vi "start_sweep.vi"(8 "error in (no error)":errorcluster, 11 "DL090430TriggeredExperimentController in":refnum<class "ExperimentControllerDL090803Triggered.lvclass">) -> (0 "error out":errorcluster, 3 "DL090430TriggeredExperimentController out":refnum<class "ExperimentControllerDL090803Triggered.lvclass">)   [LabVIEW 2010, in "ExperimentControllerDL090803Triggered.lvclass"]
uses:
  ExperimentControllerDL090803Triggered.lvclass
  ExperimentControllerDL090803Triggered.lvclass/ExperimentControllerDL090803Triggered.ctl
  DAQ/GenericDAQ/GenericDAQ/GenericDAQ.lvclass
  ScanHead/GenericScanHead/GenericScanHead/GenericScanHead.lvclass
  ImagingMode/GenericImagingMode/GenericImagingMode/GenericImagingMode.lvclass
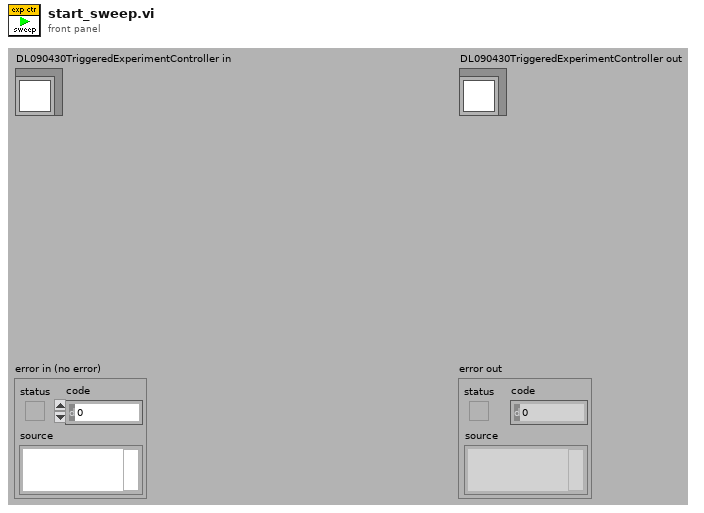
[diagram p1: front panel]
types:
  T1 = typedef "GenericToplevelComponent.lvclass/common_trigger_enum.ctl" = enum16{"NULL", "initialise", "terminate", "fetch command", "fetch data", "attach observer", "register as observer", "detach observer", "acknowledge", "start", "stop", "sweep started", "sweep finished", "experiment started", "experiment stopped"}
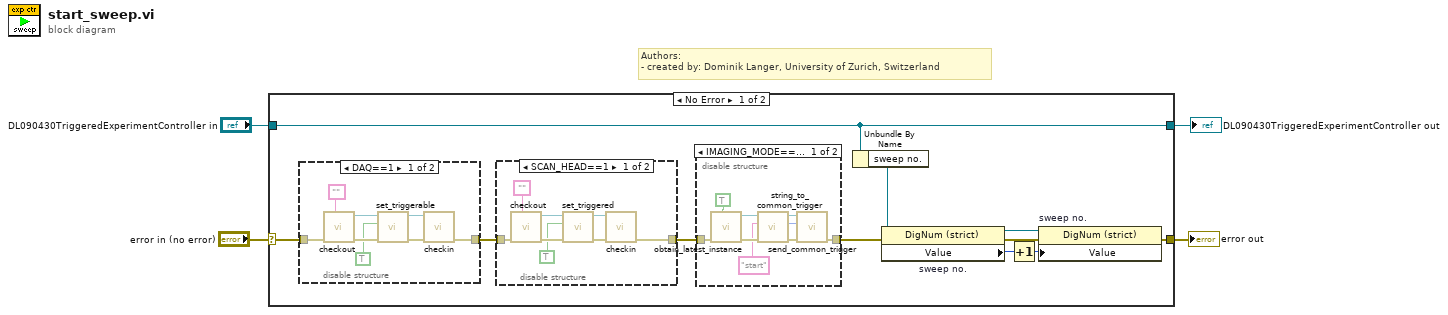
[diagram p0: block diagram]
diagram:
  # "Authors: \n- created by: Dominik Langer, University of Zurich, Switzerland"
  n1 = case shown="No Error" "error in (no error)" {
    selector: "error in (no error)" -> [w7 w45]
    tunnel: [w8 w45] -> w3
    tunnel: [w15 w44] -> w1
    tunnel: "DL090430TriggeredExperimentController in" -> [w15 w44]
    frame No Error {
      n2 = disable-structure shown="DAQ==1" {
        disable-tunnel: w7 -> [w32 w33]
        disable-tunnel: [w31 w33] -> w6
        frame condition #0 {
          n3 = call "checkout.vi"("locked by?"="", "error in (no error)"=w32) -> ("error out"=w30:errorcluster, "GenericDAQ out"=w27:refnum<class "GenericDAQ.lvclass">)  [unwired: 8 out]
          n4 = call-dynamic "set_triggerable.vi"("error in (no error)"=w30, "triggerable?"=TRUE, "GenericDAQ in"=w27) -> ("error out"=w29:errorcluster, "GenericDAQ out"=w26:refnum<class "GenericDAQ.lvclass">)  [unwired: 7 out]
          n5 = call-dynamic "checkin.vi"("error in (no error)"=w29, "GenericDAQ in"=w26) -> ("error out"=w31:errorcluster)  [unwired: 8 in, 1 out]
        }
        frame condition #1 (active) {
        }
      }
      n6 = disable-structure shown="SCAN_HEAD==1" {
        disable-tunnel: w6 -> [w23 w24]
        disable-tunnel: [w18 w24] -> w5
        frame condition #0 {
          n7 = call "checkout.vi"("locked by?"="", "error in (no error)"=w23) -> ("error out"=w22:errorcluster, "GenericScanHead out"=w20:refnum<class "GenericScanHead.lvclass">)  [unwired: 8 out]
          n8 = call-dynamic "set_triggered.vi"("error in (no error)"=w22, "triggered?"=TRUE ("triggerable?"), "GenericScanHead.lvclass in"=w20) -> ("error out"=w21:errorcluster, "GenericScanHead.lvclass out"=w19:refnum<class "GenericScanHead.lvclass">)  [unwired: 7 out]
          n9 = call-dynamic "checkin.vi"("error in (no error)"=w21, "GenericScanHead in"=w19) -> ("error out"=w18:errorcluster)  [unwired: 8 in, 1 out]
        }
        frame condition #1 (active) {
        }
      }
      n10 = disable-structure shown="IMAGING_MODE==1" {
        disable-tunnel: w5 -> [w42 w43]
        disable-tunnel: [w41 w43] -> w13
        frame condition #0 {
          n11 = call "obtain_latest_instance.vi"("quick, but maybe outdated?"=TRUE ("lock?"), "error in (no error)"=w42) -> ("error out"=w39:errorcluster, "GenericScanMode out"=w38:refnum<class "GenericImagingMode.lvclass">)  [unwired: 8 in]
          n12 = call-dynamic "string_to_common_trigger.vi"("error in (no error)"=w39, "trigger string"="start", "GenericToplevelComponent in"=w38) -> ("error out"=w36:errorcluster, "trigger"=w35:T1, "GenericToplevelComponent out"=w37:refnum<class "GenericImagingMode.lvclass">)  [unwired: 6 in]
          n13 = call-dynamic "send_common_trigger.vi"("error in (no error)"=w36, "trigger"=w35, "GenericToplevelComponent in"=w37) -> ("error out"=w41:errorcluster)  [unwired: 6 in, 2 out]
        }
        frame condition #1 (active) {
        }
      }
      n14 = Unbundle By Name(w15) -> ("sweep no."=w14:refnum<vi>)
      n15 = property on="sweep no." class="DigNum (strict)"(reference=w14, error in=w13) -> (reference out=w11:refnum<vi>, error out=w12:errorcluster, "Value"=w10:i32)
      n16 = Increment(x=w10) -> (x+1=w9:i32)
      n17 = property on="sweep no." class="DigNum (strict)"(reference=w11, error in=w12, "Value"=w9) -> (error out=w8:errorcluster)  [unwired: 1 out]
    }
    frame Error {
    }
  }
  "error out" <- w3
  "DL090430TriggeredExperimentController out" <- w1
